vi "Register to Discovery Service.vi"(0 "gRPC Client in":refnum<class "Discovery_client.lvclass">, 5 "Server Address":string, 7 "Listening Port":i32, 11 "error in (no error)":errorcluster) -> (4 "gRPC Client":refnum<class "Discovery_client.lvclass">, 6 "Response Data":T1, 15 "error out":errorcluster)   [LabVIEW 2020, in "LineRegulation.lvlib" / "MeasurementService_Template.lvclass"]
uses:
  MeasurementService_Template.lvclass
  <vilib>/gRPC/Discovery Client/Discovery_client Class/Discovery_client.lvclass
  <vilib>/gRPC/Discovery Client/Discovery_client Class/RPC Messages/NIMeasurementServices_RegisterServiceResponse/NIMeasurementServices_RegisterServiceResponse_Data.ctl
  <vilib>/gRPC/Discovery Client/Discovery_client Class/RPC Messages/NIMeasurementServices_RegisterServiceRequest/NIMeasurementServices_RegisterServiceRequest_Data.ctl
  <vilib>/gRPC/Discovery Client/Discovery_client Class/RPC Messages/NIMeasurementServices_ServiceDescriptor/NIMeasurementServices_ServiceDescriptor_Data.ctl
  <vilib>/gRPC/Discovery Client/Discovery_client Class/RPC Messages/NIMeasurementServices_ServiceLocation/NIMeasurementServices_ServiceLocation_Data.ctl
  LineRegulation.lvlib
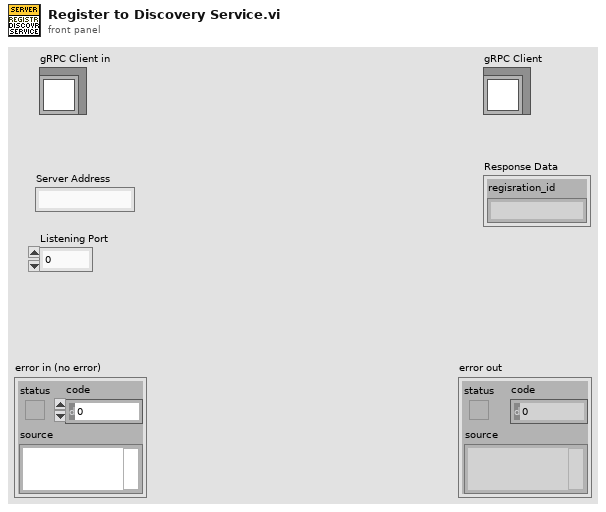
[diagram p1: front panel]
types:
  T1 = typedef "Discovery_client-release.lvlib/Discovery_client.lvclass/NIMeasurementServices_RegisterServiceResponse_Data.ctl" = cluster{"regisration_id":string}
  T2 = typedef "Discovery_client-release.lvlib/Discovery_client.lvclass/NIMeasurementServices_RegisterServiceRequest_Data.ctl" = cluster{"service_description":T3, "provided_services":string[], "location":T4}
  T3 = typedef "Discovery_client-release.lvlib/Discovery_client.lvclass/NIMeasurementServices_ServiceDescriptor_Data.ctl" = cluster{"service_id":string, "name":string, "description_url":string, "service_class":string}
  T4 = typedef "Discovery_client-release.lvlib/Discovery_client.lvclass/NIMeasurementServices_ServiceLocation_Data.ctl" = cluster{"location":string, "optimal_route":string, "insecure_port":string, "ssl_authenticated_port":string}
  T5 = typedef "LineRegulation.lvlib/MeasurementService_Template.lvclass/Measurement_v1_MeasurementDetails_Data.ctl" = cluster{"display_name":string, "version":string, "measurement_type":string, "product_type":string}
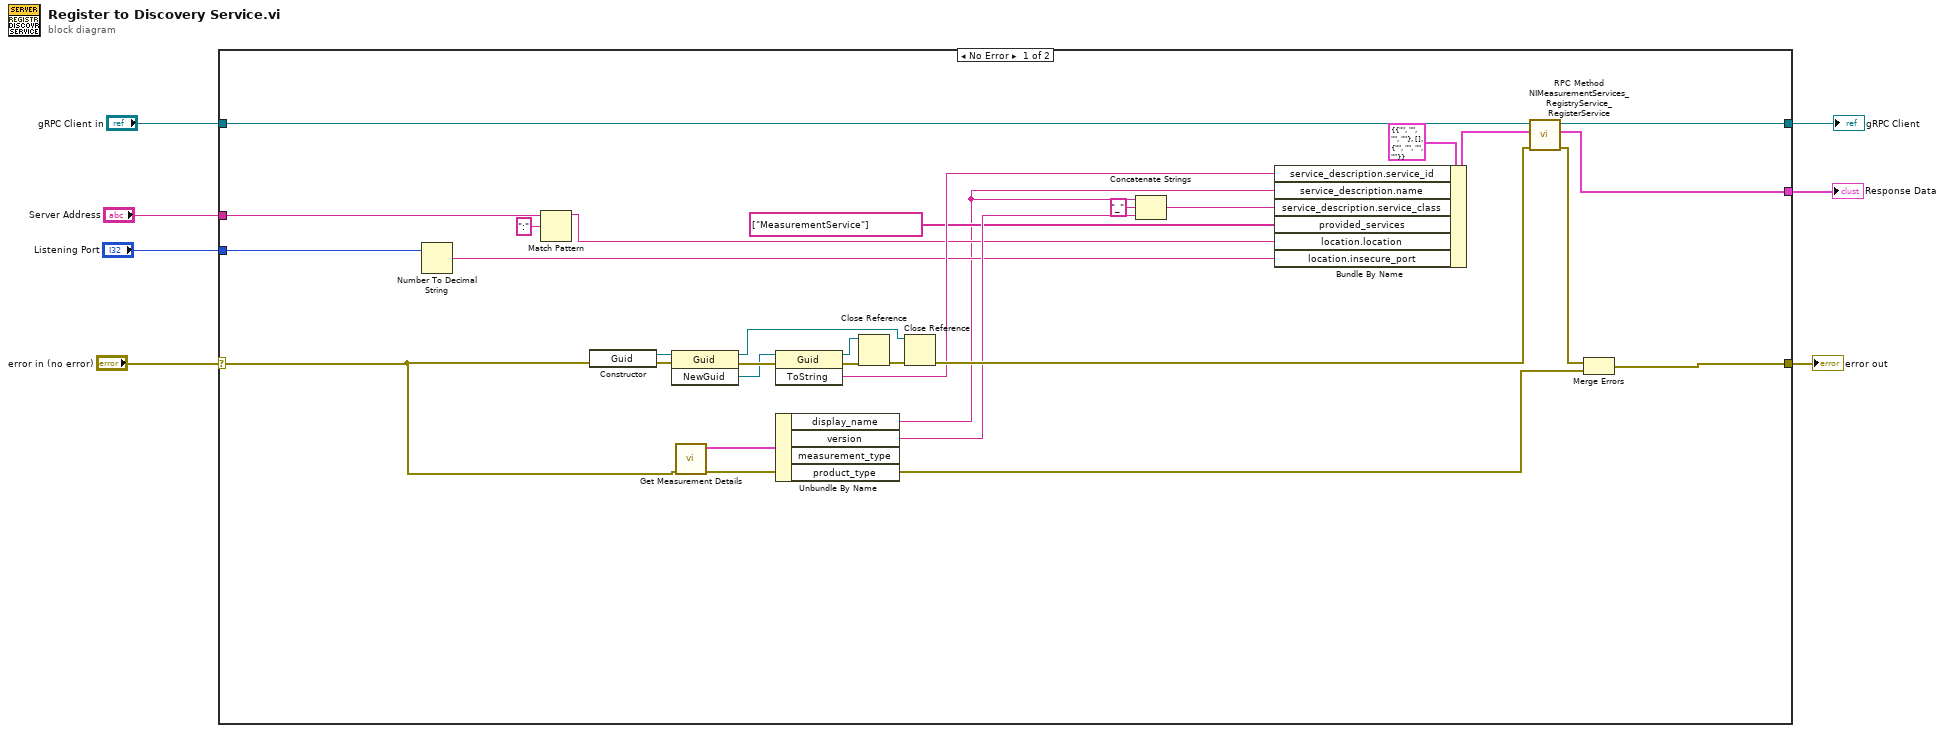
[diagram p0: block diagram]
diagram:
  n1 = case shown="No Error" "error in (no error)" {
    selector: "error in (no error)" -> [w9 w39]
    tunnel: [w13 w39] -> w6
    tunnel: "gRPC Client in" -> [w16 w38]
    tunnel: [w15 w38] -> w4
    tunnel: [w14 _] -> w3
    tunnel: "Listening Port" -> [w12 _]
    tunnel: "Server Address" -> [w11 _]
    frame No Error {
      n2 = Number To Decimal String(number=w12) -> (decimal integer string=w21:string)  [unwired: 1 in]
      n3 = Match Pattern(string=w11, regular expression=":") -> (before substring=w19:string)  [unwired: 1 in, 3 out]
      n4 = constructor class="Guid"(error in=w9) -> (reference out=w29:refnum<k24>, error out=w28:errorcluster)  [unwired: 2 in, 1 out]
      n5 = invoke class="Guid" method="NewGuid"(reference=w29, error in=w28) -> (reference out=w35:refnum<k24>, error out=w32:errorcluster, "NewGuid"=w30:refnum<k24>)  [unwired: 1 in]
      n6 = call "Get Measurement Details.vi"("error in"=w9) -> ("error out"=w8:errorcluster, "measurement_details"=w10:T5)  [unwired: 9 in]
      n7 = invoke class="Guid" method="ToString"(reference=w30, error in=w32) -> (reference out=w33:refnum<k24>, error out=w31:errorcluster, "ToString"=w26:string)  [unwired: 1 in]
      n8 = Unbundle By Name(w10) -> ("display_name"=w17:string, "version"=w25:string)  [unwired: 2 out]
      n9 = Close Reference(reference=w33, error in (no error)=w31) -> (error out=w34:errorcluster)
      n10 = Close Reference(reference=w35, error in (no error)=w34) -> (error out=w27:errorcluster)
      n11 = Concatenate Strings(w17, "_" ("string"), w25) -> (w18:string)
      n12 = Bundle By Name(cluster=T2 {"service_description"={"service_id"="", "name"="", "description_url"="", "service_class"=""}, "provided_services"=[], "location"={"location"="", "optimal_route"="", "insecure_port"="", "ssl_authenticated_port"=""}} ("Request Data"), "service_description.service_id"=w26, "service_description.name"=w17, "service_description.service_class"=w18, "provided_services"=string[] ["MeasurementService"], "location.location"=w19, "location.insecure_port"=w21) -> (w22:T2)
      n13 = call <vilib>:"RPC Method NIMeasurementServices_RegistryService_RegisterService.vi"("error in (no error)"=w27, "Request Data"=w22, "gRPC Client in"=w16) -> ("error out"=w36:errorcluster, "Response Data"=w14:T1, "gRPC Client out"=w15:refnum<class "Discovery_client.lvclass">)  [unwired: 6 in]
      n14 = Merge Errors(w36, w8) -> (w13:errorcluster)
    }
    frame Error {
    }
  }
  "error out" <- w6
  "gRPC Client" <- w4
  "Response Data" <- w3
